vi "Load Bitmap.vi"(8 "error in":errorcluster, 11 "File":string="c:\\temp\\hello.bmp") -> (0 "error out":errorcluster, 3 "Surface Pointer":u32 format="%.0x")   [LabVIEW 2014, in "LibSDL2.lvlib"]
uses:
  LibSDL2.lvlib
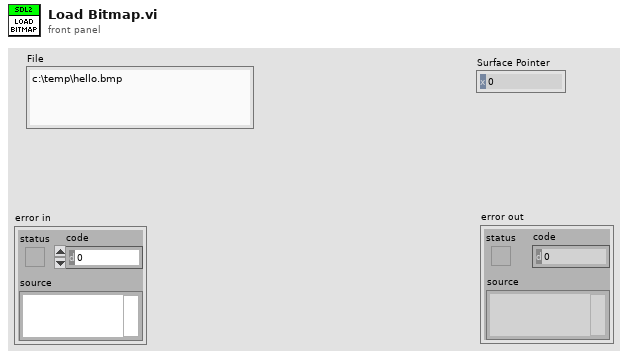
[diagram p1: front panel]
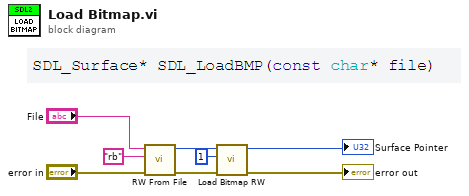
[diagram p0: block diagram]
diagram:
  n1 = call "RW From File.vi"("error in"="error in", "Mode"="rb", "File"="File") -> ("error out"=w5:errorcluster, "RWops Pointer"=w4:u32)  [unwired: 7 in]
  n2 = call "Load Bitmap RW.vi"("error in"=w5, "Free Source"=1, "RWops Source Pointer"=w4) -> ("error out"=→"error out":errorcluster, "Surface Pointer"=→"Surface Pointer":u32)  [unwired: 7 in]
